vi "servo motor.vi"() -> ()   [LabVIEW 2017]
uses:
  <vilib>/MakerHub/LINX/Public/Utilities/Open Serial.vi
  <vilib>/MakerHub/LINX/Public/Sensors/Motion/Servo/Servo Open N Channels.vi
  <vilib>/MakerHub/LINX/Public/Sensors/Motion/Servo/Servo Set Pulse Width N Channels.vi
  <vilib>/MakerHub/LINX/Public/Sensors/Motion/Servo/Servo Close N Channels.vi
  <vilib>/MakerHub/LINX/LMH-LINX.lvlib
  <vilib>/MakerHub/LINX/Public/Sensors/Motion/Servo/Servo.lvlib
panel:
  in  "Serial Port":refnum<visa-resource-name>="COM8"
  in  "stop":bool
  out "Loop Rate (Hz)":u32
  in  "Array":T1(array[cluster])=[{"Position (uS)"=1500, "Servo Channel"=11}, {"Position (uS)"=1500, "Servo Channel"=9}, {"Position (uS)"=1500, "Servo Channel"=6}, {"Position (uS)"=1500, "Servo Channel"=4}, {"Position (uS)"=1500, "Servo Channel"=12}] {"Position (uS)" min=500 max=2500 step=1 scale=500.0..2500.0}
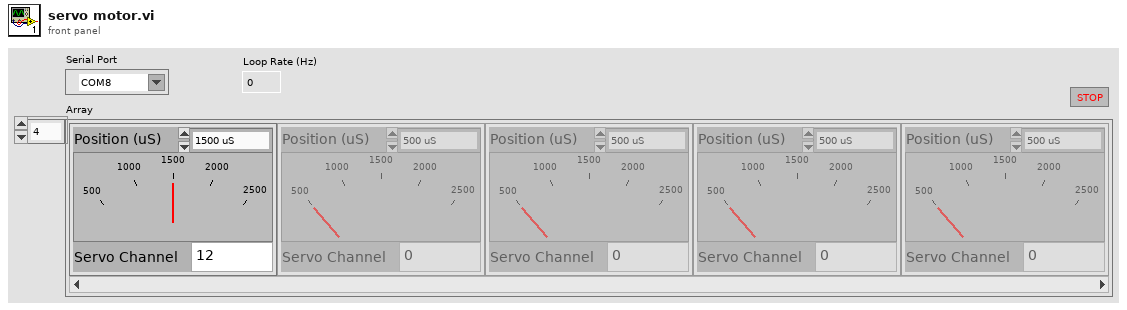
[diagram p1: front panel]
types:
  T1 = cluster{"Position (uS)":u16, "Servo Channel":u8}[]
  T2 = typedef "LMH-LINX.lvlib/LINX Ref.ctl" = cluster{"IO":T3, "Interface":T4, "LINX Device Config":T5}
  T3 = typedef "LMH-LINX.lvlib/Platform.ctl" = enum16{"Remote", "Local"}
  T4 = typedef "LMH-LINX.lvlib/Interface.ctl" = enum16{"Serial", "TCP"}
  T5 = typedef "LMH-LINX.lvlib/Device.lvlib/LINX Device Config.ctl" = cluster{"Interface":T4, "COM Port":refnum<visa-resource-name>, "TCP Configuration":T6, "Device Family":u8, "Device ID":u8, "Device Name":string, "TCP Ref":refnum<k5>, "Channels":T7}
  T6 = typedef "LMH-LINX.lvlib/Device.lvlib/TCP Config.ctl" = cluster{"IP Address":string, "Port":u16}
  T7 = typedef "LMH-LINX.lvlib/Channels.ctl" = cluster{"DI":u8[], "DO":u8[], "AI":u8[], "AO":u8[], "PWM":u8[], "QE":u8[], "UART":u8[], "I2C 2":u8[], "SPI":u8[], "CAN":u8[], "Servo":u8[], "AI Ref (V)":dbl, "AI Resolution (Bits)":u8, "AO Ref (V)":dbl, "AO Resolution (Bits)":u8}
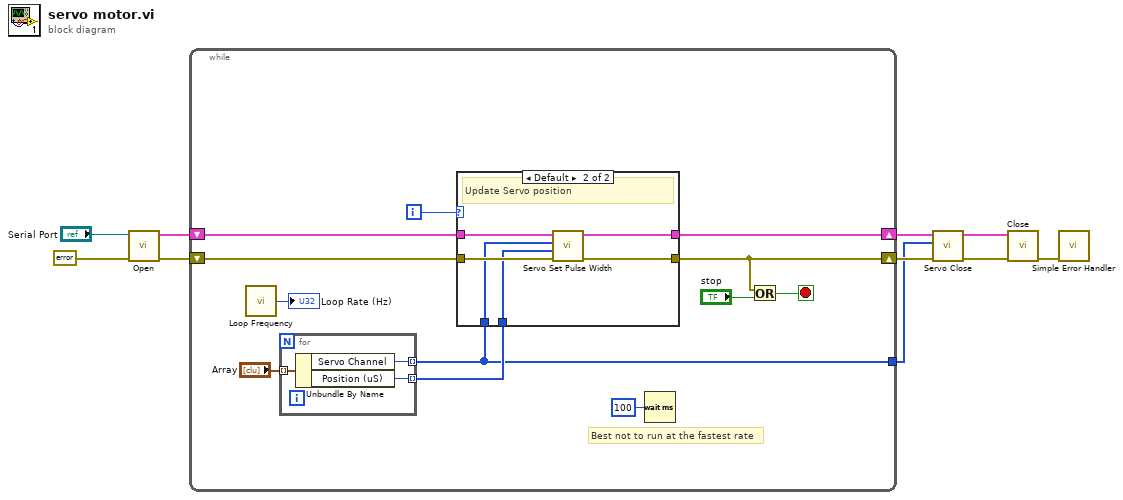
[diagram p0: block diagram]
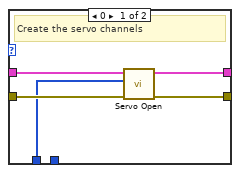
[diagram p2: hidden frame]
diagram:
  n1 = call-poly <vilib>:"Open.vi"("Error In"=errorcluster {"status"=FALSE, "code"=0, "source"=""}, "Serial Port"="Serial Port") -> ("Error Out"=w3:errorcluster, "LINX Resource"=w8:T2)  [unwired: 7 in, 1 out]
  n2 = while {
    shift-right: [w21] -> w7
    shift-left: w8 -> [w22]
    shift-right: [w18] -> w4
    shift-left: w3 -> [w20]
    tunnel: [w12] -> w1
    i -> [w15]
    stop <- w16 stop-if-true
    # "Best not to run at the fastest rate"
    n3 = call <vilib>:"Loop Frequency.vi"() -> ("Loop Rate (Hz)"=→"Loop Rate (Hz)":u32)
    n4 = for {
      tunnel: "Array" -> [w25] mode=indexing
      tunnel: [w24] -> w12 mode=indexing
      tunnel: [w23] -> w13 mode=indexing
      n5 = Unbundle By Name(w25) -> ("Servo Channel"=w24:u8, "Position (uS)"=w23:u16)
    }
    n6 = case shown="Default" w15 {
      tunnel: w22 -> [w30 w36]
      tunnel: [w28 w35] -> w21
      tunnel: w20 -> [w29 w34]
      tunnel: [w27 w33] -> w18
      tunnel: w12 -> [w26 w32]
      tunnel: w13 -> [_ w31]
      frame 0 {
        # "Create the servo channels"
        n7 = call-poly <vilib>:"Servo Open.vi"("Error In"=w29, "Servo Channels"=w26, "LINX Resource"=w30) -> ("Error Out"=w27:errorcluster, "LINX Resource"=w28:T2)  [unwired: 7 in]
      }
      frame Default {
        # "Update Servo position"
        n8 = call-poly <vilib>:"Servo Set Pulse Width.vi"("Error In"=w34, "Pulse Widths (uS)"=w31, "Servo Channels"=w32, "LINX Resource"=w36) -> ("Error Out"=w33:errorcluster, "LINX Resource"=w35:T2)  [unwired: 6 in]
      }
    }
    n9 = Wait (ms)(milliseconds to wait=u32 100) -> ()  [unwired: 1 out]
    n10 = Or(x=w18, y="stop") -> (x .or. y?=w16:bool)
  }
  n11 = call-poly <vilib>:"Servo Close.vi"("Error In"=w4, "Servo Channels"=w1, "LINX Resource"=w7) -> ("Error Out"=w5:errorcluster, "LINX Resource"=w6:T2)  [unwired: 7 in]
  n12 = call <vilib>:"Close.vi"("Error In"=w5, "LINX Resource"=w6) -> ("Error Out"=w10:errorcluster)  [unwired: 9 in]
  n13 = call <vilib>:"Simple Error Handler.vi"("error in (no error)"=w10) -> ()  [unwired: 4 in, 5 out]
